vi "S2C_ExeBuildScript.vi"(8 "Error In":errorcluster, 11 "Entry":string) -> (0 "Error Out":errorcluster, 3 "Data":string[][](array[string]))   [LabVIEW 2015]
doc: "Converts a script line entry into an executable table entry."
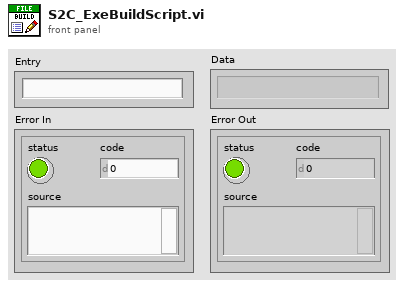
[diagram p1: front panel]
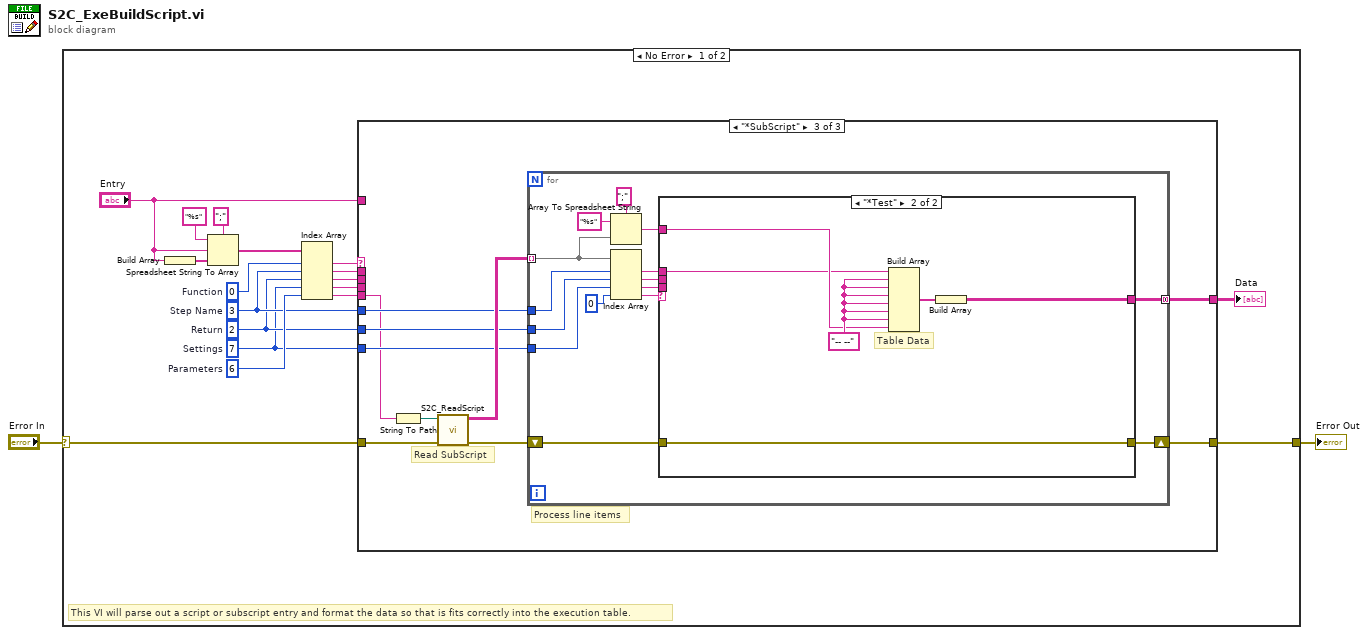
[diagram p0: block diagram]
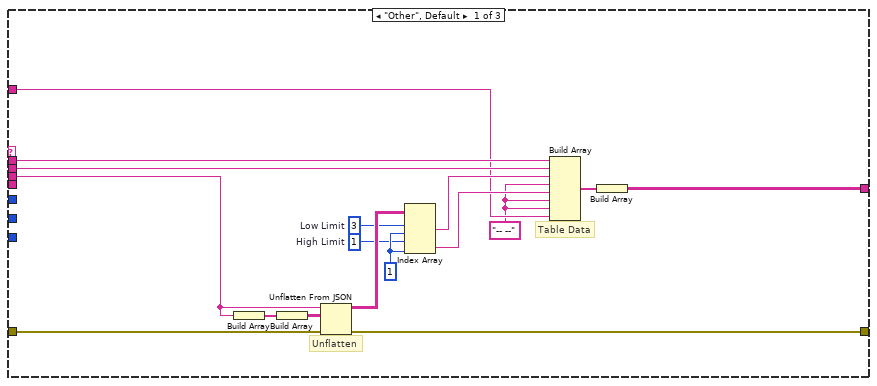
[diagram p2: hidden frame]
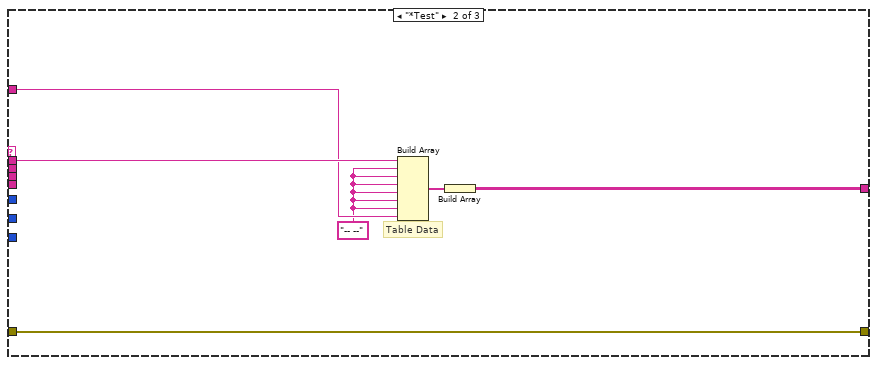
[diagram p3: hidden frame]
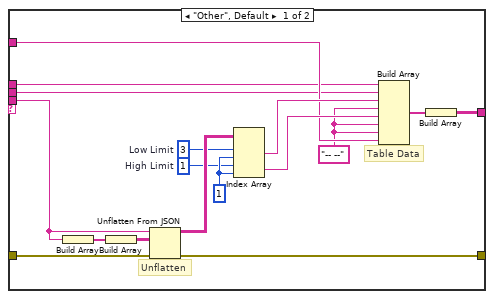
[diagram p4: hidden frame]
diagram:
  n1 = case shown="No Error" "Error In" {
    selector: "Error In" -> [w16 w92]
    tunnel: [w14 w92] -> w1
    frame No Error {
      w7 = 6  # Parameters
      w12 = 0  # Function
      w3 = 7  # Settings
      w4 = 2  # Return
      w5 = 3  # Step Name
      # "This VI will parse out a script or subscript entry and format the data so that is fits correctly into the execution table."
      n2 = Build Array("Entry") -> (w18:string[])
      n3 = Spreadsheet String To Array(delimiter (Tab)=";", format string="%s", spreadsheet string="Entry", array type (2D Dbl)=w18) -> (array=w17:string[])
      n4 = Index Array(array=w17, index #1=w12, index #2=w5, index #3=w4, index #4=w3, index #5=w7) -> (element #1=w11:string, element #2=w10:string, element #3=w9:string, element #4=w8:string, element #5=w6:string)
      n5 = case shown="\"*SubScript\"" w11 {
        tunnel: w16 -> [w37 w38 w53]
        tunnel: w8 -> [w36 _ _]
        tunnel: w10 -> [w29 w43 _]
        tunnel: w9 -> [w28 _ _]
        tunnel: [w25 w41 w46] -> w15
        tunnel: [w24 w38 w51] -> w14
        tunnel: "Entry" -> [w22 w40 _]
        tunnel: w6 -> [_ _ w45]
        tunnel: w5 -> [_ _ w49]
        tunnel: w4 -> [_ _ w48]
        tunnel: w3 -> [_ _ w47]
        frame "Other", Default {
          w21 = "-- --"
          w30 = 1  # High Limit
          w32 = 3  # Low Limit
          w31 = 1 ("disabled index (col)")
          # "Table Data"
          # "Unflatten"
          n6 = Build Array(w36) -> (w35:string[])
          n7 = Build Array(w35) -> (w34:string[][])
          n8 = Unflatten From JSON(JSON string=w36, type and defaults=w34, error in (no error)=w37) -> (value=w33:string[][], error out=w24:errorcluster)  [unwired: 4 in]
          n9 = Index Array(array=w33, index (row) #1=w32, index (col) #1=w31, index (row) #2=w30, index (col) #2=w31) -> (element #1=w27:string, element #2=w23:string)
          n10 = Build Array(w29, w28, w27, w21, w23, w21, w21, w22) -> (w26:string[])
          n11 = Build Array(w26) -> (w25:string[][])
        }
        frame "*Test" {
          w39 = "-- --"
          # "Table Data"
          n12 = Build Array(w43, w39, w39, w39, w39, w39, w39, w40) -> (w42:string[])
          n13 = Build Array(w42) -> (w41:string[][])
        }
        frame "*SubScript" {
          # "Process line items"
          # "Read SubScript"
          n14 = String To Path(string=w45) -> (path=w44:path)
          n15 = call "S2C_ReadScript.vi"("Error In"=w53, "FilePath"=w44) -> ("Error Out"=w52:errorcluster, "Data"=w50:string[][])  [unwired: 8 in]
          n16 = for {
            shift-right: [w67] -> w51
            shift-left: w52 -> [w68]
            tunnel: w50 -> [w63] mode=indexing
            tunnel: w49 -> [w66]
            tunnel: w48 -> [w65]
            tunnel: w47 -> [w64]
            tunnel: [w58] -> w46 mode=concatenating
            n17 = Array To Spreadsheet String(delimiter (Tab)=";", array=w63, 3:"%s" ("format string")) -> (spreadsheet string=w61:string)
            n18 = Index Array(array=w63, index #1=w66, index #2=w65, index #3=w64, index #4=0 ("index")) -> (element #1=w56:string, element #2=w59:string, element #3=w60:string, element #4=w54:string)
            n19 = case shown="\"*Test\"" w54 {
              tunnel: w68 -> [w76 w87]
              tunnel: [w75 w87] -> w67
              tunnel: w61 -> [w74 w89]
              tunnel: w60 -> [w73 _]
              tunnel: w59 -> [w72 _]
              tunnel: [w71 w88] -> w58
              tunnel: w56 -> [w69 w86]
              frame "Other", Default {
                w70 = "-- --"
                w80 = 1  # High Limit
                w82 = 3  # Low Limit
                w81 = 1 ("disabled index (col)")
                # "Table Data"
                # "Unflatten"
                n20 = Build Array(w73) -> (w85:string[])
                n21 = Build Array(w85) -> (w84:string[][])
                n22 = Unflatten From JSON(JSON string=w73, type and defaults=w84, error in (no error)=w76) -> (value=w83:string[][], error out=w75:errorcluster)  [unwired: 4 in]
                n23 = Index Array(array=w83, index (row) #1=w82, index (col) #1=w81, index (row) #2=w80, index (col) #2=w81) -> (element #1=w79:string, element #2=w77:string)
                n24 = Build Array(w69, w72, w79, w70, w77, w70, w70, w74) -> (w78:string[])
                n25 = Build Array(w78) -> (w71:string[][])
              }
              frame "*Test" {
                w90 = "-- --"
                # "Table Data"
                n26 = Build Array(w86, w90, w90, w90, w90, w90, w90, w89) -> (w91:string[])
                n27 = Build Array(w91) -> (w88:string[][])
              }
            }
          }
        }
      }
      "Data" <- w15
    }
    frame Error {
    }
  }
  "Error Out" <- w1
